vi "Calibrate Ticks 2 Volts (uSMC).vi"(8 "error in (no error)":errorcluster, 10 "Case":i32, 11 "VoltageTicks":u16) -> (0 "error out":errorcluster, 3 "VoltageVolts":dbl)   [LabVIEW 2010, in "SignalWriterMH110203USBStepperMotor.lvclass"]
uses:
  SignalWriterMH110203USBStepperMotor.lvclass
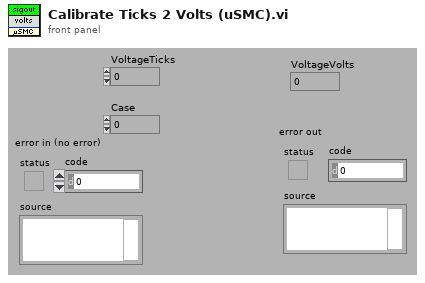
[diagram p1: front panel]
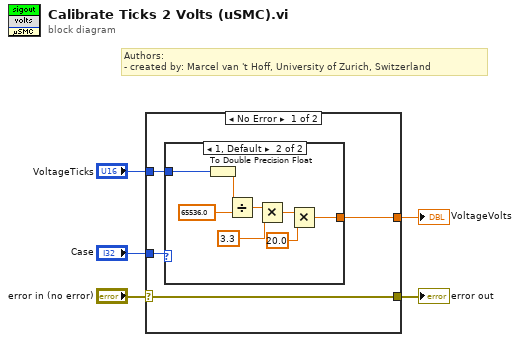
[diagram p0: block diagram]
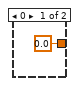
[diagram p2: hidden frame]
diagram:
  # "Authors: \n- created by: Marcel van 't Hoff, University of Zurich, Switzerland"
  n1 = case shown="No Error" "error in (no error)" {
    selector: "error in (no error)" -> [w7 w19]
    tunnel: "Case" -> [w9 _]
    tunnel: "VoltageTicks" -> [w8 _]
    tunnel: [w7 w19] -> w2
    tunnel: [w6 _] -> w1
    frame No Error {
      n2 = case shown="1, Default" w9 {
        tunnel: w8 -> [_ w18]
        tunnel: [0.0 ("VoltageTicks") w11] -> w6
        frame 0 {
        }
        frame 1, Default {
          n3 = To Double Precision Float(number=w18) -> (double precision float=w17:dbl)
          n4 = Divide(x=w17, y=65536.0) -> (x/y=w15:dbl)
          n5 = Multiply(x=w15, y=3.3) -> (x*y=w13:dbl)
          n6 = Multiply(x=w13, y=20.0) -> (x*y=w11:dbl)
        }
      }
    }
    frame Error {
    }
  }
  "error out" <- w2
  "VoltageVolts" <- w1
